vi "NG Pack量測值轉換.vi"(7 "位數":i32=9, 8 "error in (no error)":errorcluster, 9 "input string":string, 10 "PLC address":i32=20, 11 "Input Data":dbl=222.33) -> (0 "error out":errorcluster, 3 "Array":u16[](array[numeric]))   [LabVIEW 2019]
uses:
  Ctrl/ModbusCmd.ctl
panel:
  out "x+y":i32
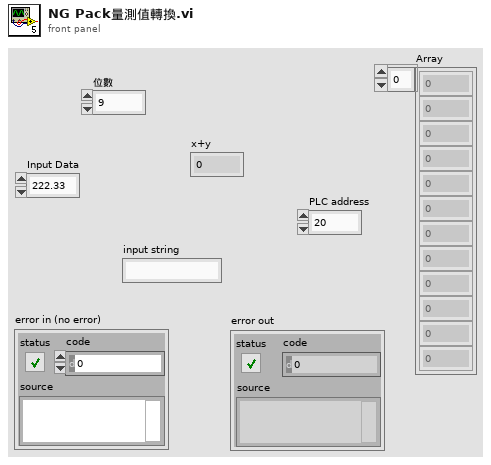
[diagram p1: front panel]
types:
  T1 = cluster{"starting address":u16, "number of inputs":u16, "Sat Coils":bool[], "Holding Registers":u16[]}
  T2 = typedef "ModbusCmd.ctl" = enum16{"Connect", "Disconnect", "Init", "Fetch Basic Objects", "Fetch Input Refisters", "Fetch Discrete Inputs", "Set Coils", "Set Holding Registers", "Write Single Holding", "Exit"}
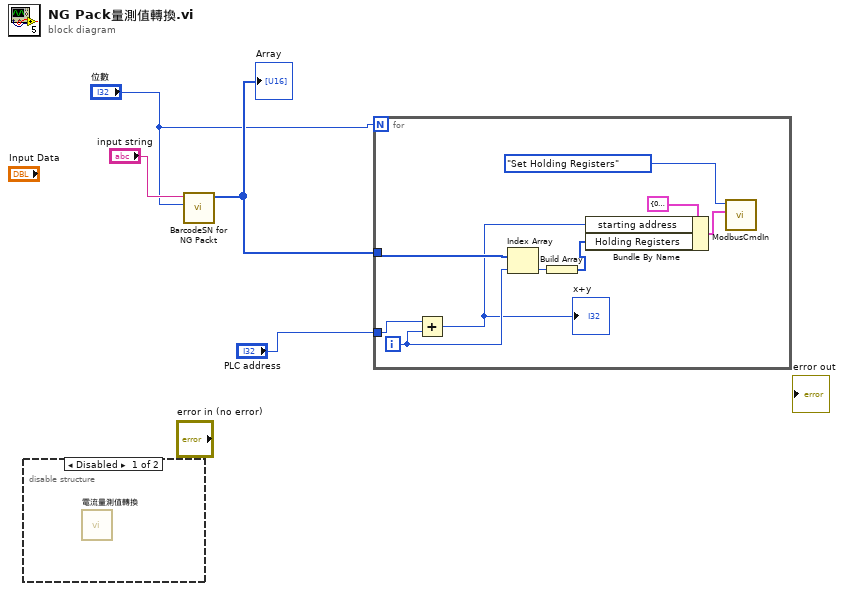
[diagram p0: block diagram]
diagram:
  n1 = disable-structure shown="Disabled" {
    frame Disabled {
      n2 = call "電流量測值轉換.vi"() -> ()  [unwired: 10 in, 2 out]
    }
    frame Enabled {
    }
  }
  n3 = call "BarcodeSN for NG Packt.vi"("位數"="位數", "String Input"="input string") -> ("Array"=w2:u16[])  [unwired: 9 in]
  "Array" <- w2
  n4 = for {
    N: "位數" -> [_]
    tunnel: w2 -> [w13]
    tunnel: "PLC address" -> [w6]
    i -> [w12]
    n5 = Add(x=w6, y=w12) -> (x+y=w11:i32)
    "x+y" <- w11
    n6 = Index Array(array=w13, index=w12) -> (element=w7:u16)
    n7 = Build Array(w7) -> (w5:u16[])
    n8 = Bundle By Name(cluster=T1 {"starting address"=0, "number of inputs"=0, "Sat Coils"=[FALSE], "Holding Registers"=[]} ("data"), "starting address"=w11, "Holding Registers"=w5) -> (w8:T1)
    n9 = call "ModbusCmdIn.vi"("data"=w8, "Enum"=ModbusCmd."Set Holding Registers") -> ()  [unwired: 9 in, 1 out]
  }
